vi "test-state-space-util--XXX.vi"() -> (3 "All Tests Passed":bool)   [LabVIEW 2019]
uses:
  <vilib>/Analysis/Matrix/Datatypes/RealMatrix.ctl
  <vilib>/Analysis/baseanly.llb/Real A x B.vi
  <vilib>/Rock Robotics/WPI/ThirdParty/JAS_Junk/TrajLib/MatBuilder_Create.vi
  <vilib>/Analysis/7linalg.llb/Transpose Matrix.vi
  <vilib>/Analysis/7linalg.llb/Real Transpose Matrix.vi
  <vilib>/Rock Robotics/WPI/ThirdParty/JAS_Junk/TrajLib/MatrixHelper_CoerceSize.vi
  <vilib>/Rock Robotics/WPI/ThirdParty/JAS_Junk/TrajLib/Matrix_Ident.vi
  <vilib>/Analysis/Matrix/Numeric/Multiply/Multiply.vi
  <vilib>/Analysis/Matrix/Numeric/Multiply/Multiply - RM,R.vi
  <vilib>/Rock Robotics/WPI/ThirdParty/JAS_Junk/TrajLib/Matrix_Exp.vi
  <vilib>/Rock Robotics/WPI/ThirdParty/JAS_Junk/TrajLib/Matrix_AssignBlock.vi
  <vilib>/Rock Robotics/WPI/ThirdParty/JAS_Junk/TrajLib/Matrix_ExtractFrom.vi
  <vilib>/Analysis/7linalg.llb/Create Special Matrix.vi
  <vilib>/Analysis/7linalg.llb/Create Special Real Matrix.vi
  <vilib>/Analysis/Matrix/Numeric/Add/Add - RM,RM.vi
  <vilib>/Analysis/Matrix/Comparison/Equal/Equal - RM,RM.vi
  <vilib>/Rock Robotics/WPI/ThirdParty/JAS_Junk/TrajLib/Trajectory_Library.lvlib
  <vilib>/Analysis/NI_AALBase.lvlib
  <vilib>/Analysis/Matrix/NI_Matrix.lvlib
panel:
  out "A+B Should be":T1
  out "A + B":T1
  out "Test x passed":bool
  out "Test 3 passed":bool
  out "Test Passed 2":bool
  out "Test Passed 1":bool
  out "Test Passed 0":bool
  out "AQ Passed":bool
  out "AQ - DiscQ":T1
  out "AQ - DiscA":T1
  out "AB-Taylor-Passed":bool
  out "ABTaylor-DiscB":T1
  out "ABTaylor - DiscA":T1
  out "AB-passed":bool
  out "AB-DiscB":T1
  out "AB - DiscA":T1
  out "x1-Disc":T1
  out "DiscA Error":bool
  out "DiscA":T1
  out "Cost Mat":T1
  out "CoVar Mat":T1
  # "1.0,   0.0,    0.0\n\n0.0,     4.0,   0.0, ;\n\n0.0,     0.0,  9.0;"
  # "1.0,      0.0,      0.0, \n\n0.0,   1.0 / 4.0,   0.0, \n\n0.0,       0.0,      1.0 / 9.0,"
  # "VecBuilder.fill(\n          x0.get(0, 0) + 1.0 * x0.get(1, 0), \n          x0.get(1, 0));"
  # "2,\n1"
  # "x0.get(0, 0) + x0.get(1, 0) + 0.5 * u.get(0, 0), \n\nx0.get(0, 0) + u.get(0, 0))"
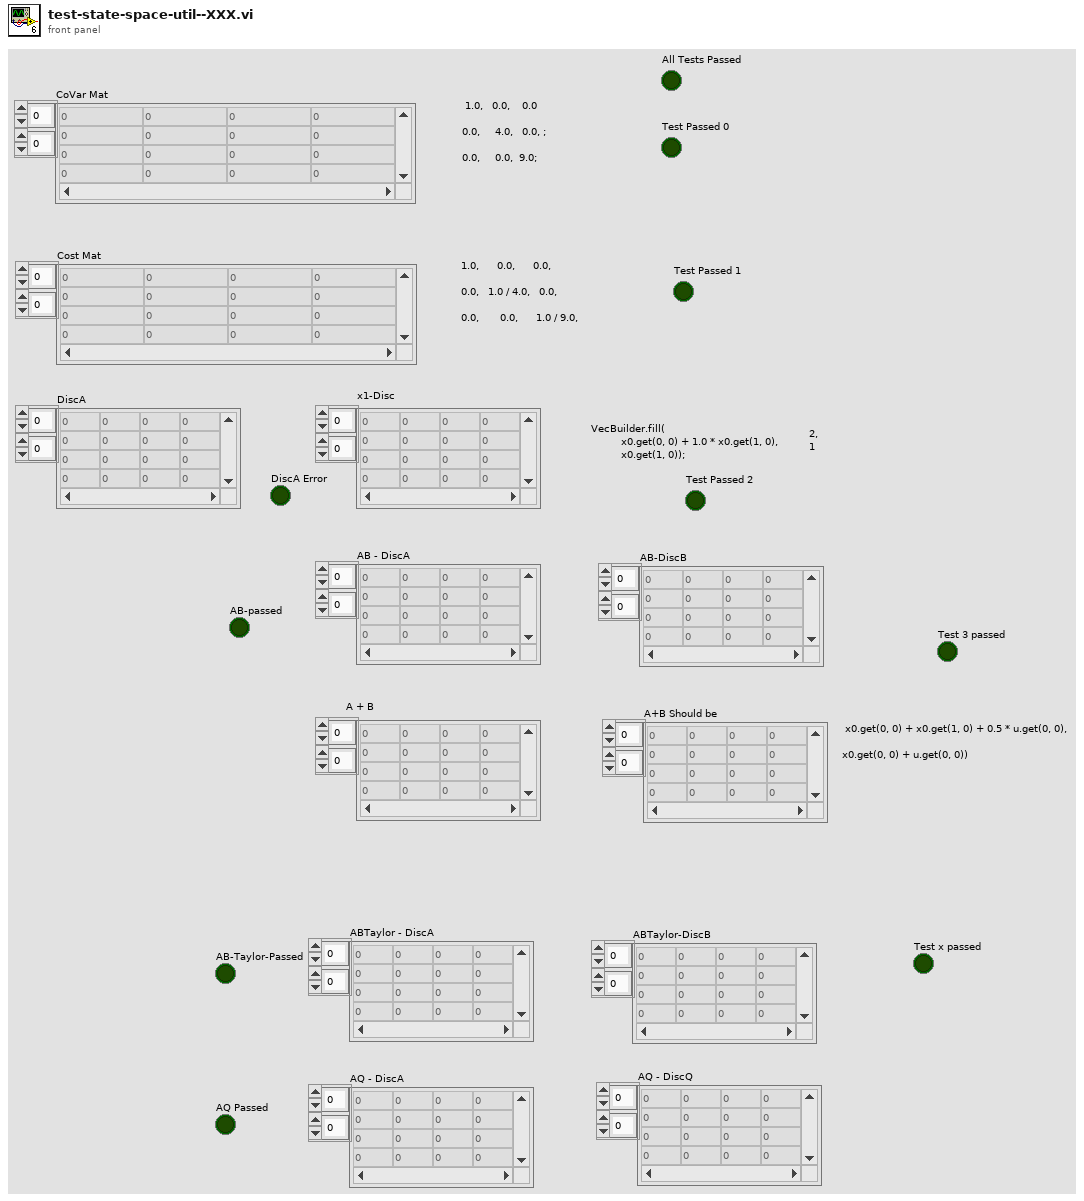
[diagram p1: front panel]
types:
  T1 = typedef "NI_Matrix.lvlib/RealMatrix.ctl" = dbl[][]
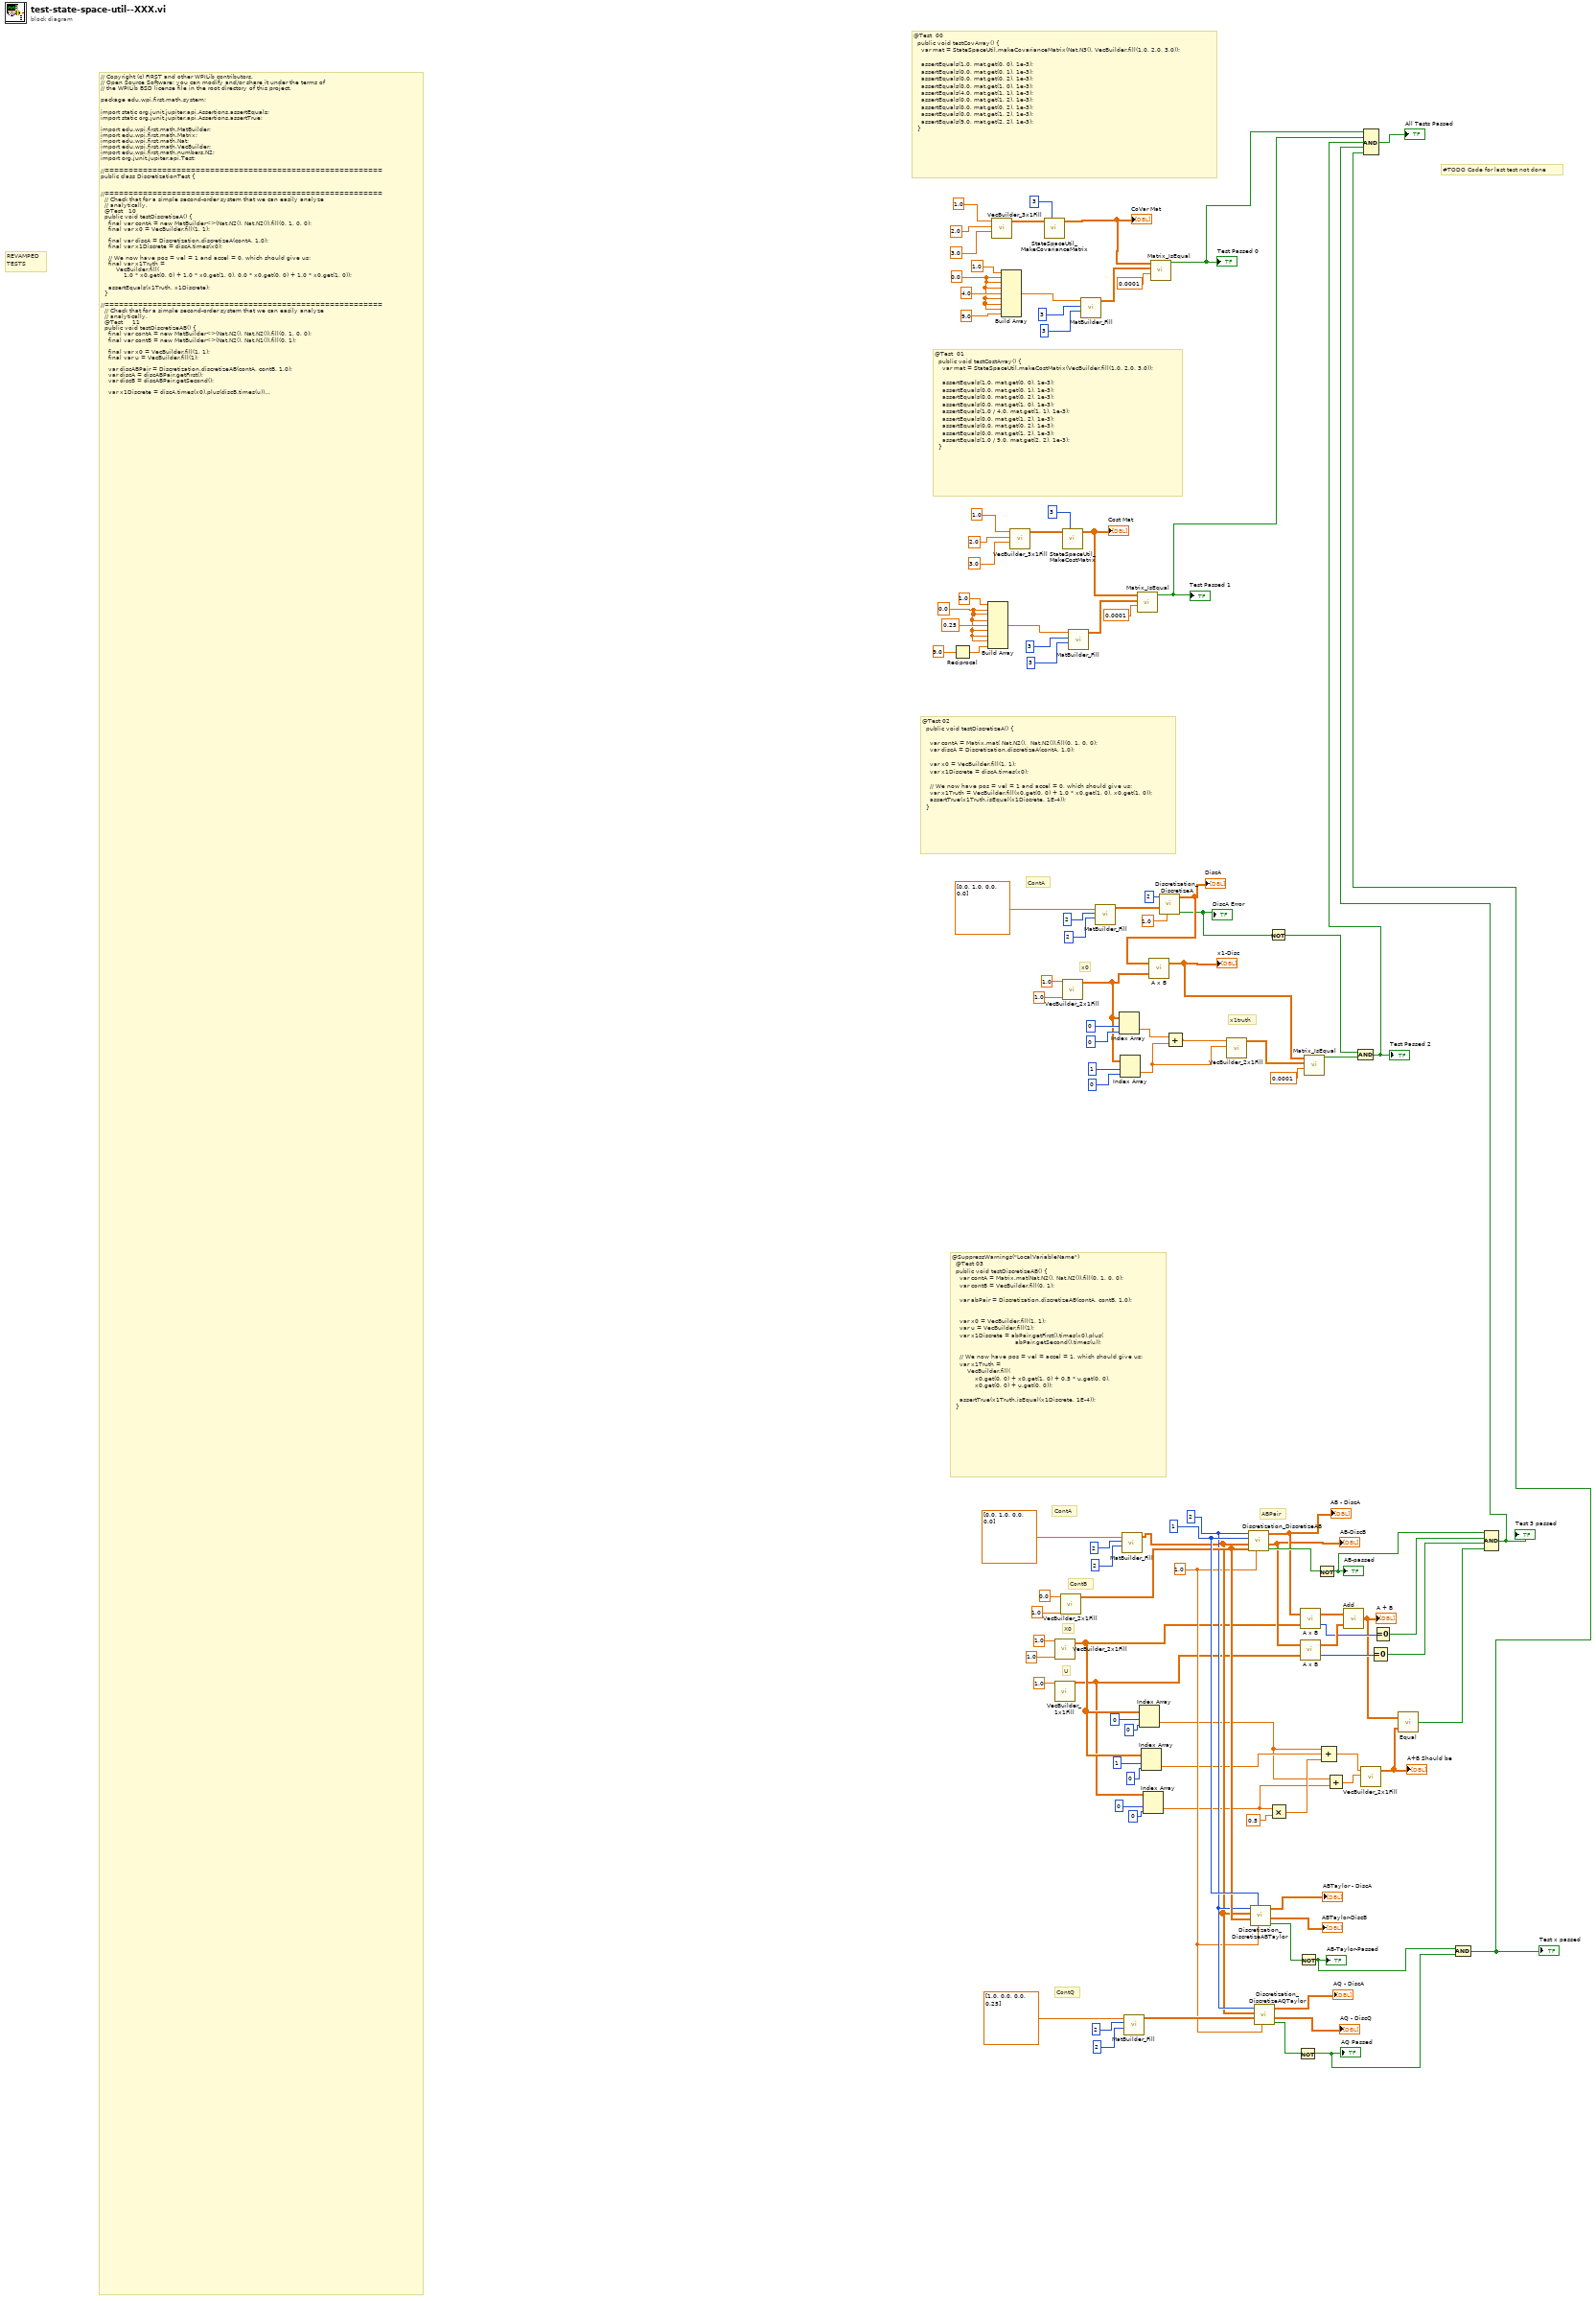
[diagram p0: block diagram]
diagram:
  w61 = 0.0 ("element")
  w71 = 0.0 ("element")
  w79 = 1.0 ("dT_Seconds")
  w89 = 1 ("Inputs")
  w82 = 2 ("States")
  # "REVAMPED\nTESTS"
  # "// Copyright (c) FIRST and other WPILib contributors.\n// Open Source Software; you can modify and/or share it under the terms of\n// the WPILib BSD license file in the root directory of this project.\n\npackage edu.wpi.first.math.system;\n\nimport static org.junit.jupiter.api.Assertions.assertEquals;\nimport static org.junit.jupiter.api.Assertions.assertTrue;\n\nimport edu.wpi.first.math.MatBuilder;\nimport edu.wpi.first.math.Matrix;\nimport edu.wpi.first.math.Nat;\nimport edu.wpi.first.math.VecBuilder;\nimport edu.wpi.first.math.numbers.N2;\nimport org.junit.jupiter.api.Test;\n\n//==========================================================\npublic class DiscretizationTest {\n\n\n//==========================================================\n  // Check that for a simple second-order system that we can easily analyze\n  // analytically,\n  @Test   10\n  public void testDiscretizeA() {\n    final var contA = new MatBuilder<>(Nat.N2(), Nat.N2()).fill(0, 1, 0, 0);\n    final var x0 = VecBuilder.fill(1, 1);\n\n    final var discA = Discretization.discretizeA(contA, 1.0);\n    final var x1Discrete = discA.times(x0);\n\n    // We now have pos = vel = 1 and accel = 0, which should give us:\n    final var x1Truth =\n        VecBuilder.fill(\n            1.0 * x0.get(0, 0) + 1.0 * x0.get(1, 0), 0.0 * x0.get(0, 0) + 1.0 * x0.get(1, 0));\n\n    assertEquals(x1Truth, x1Discrete);\n  }\n\n//==========================================================\n  // Check that for a simple second-order system that we can easily analyze\n  // analytically,\n  @Test     11\n  public void testDiscretizeAB() {\n    final var contA = new MatBuilder<>(Nat.N2(), Nat.N2()).fill(0, 1, 0, 0);\n    final var contB = new MatBuilder<>(Nat.N2(), Nat.N1()).fill(0, 1);\n\n    final var x0 = VecBuilder.fill(1, 1);\n    final var u = VecBuilder.fill(1);\n\n    var discABPair = Discretization.discretizeAB(contA, contB, 1.0);\n    var discA = discABPair.getFirst();\n    var discB = discABPair.getSecond();\n\n    var x1Discrete = discA.times(x0).plus(discB.times(u));\n\n    // We now have pos = vel = accel = 1, which should give us:\n    final var x1Truth =\n        VecBuilder.fill(\n            1.0 * x0.get(0, 0) + 1.0 * x0.get(1, 0) + 0.5 * u.get(0, 0),\n            0.0 * x0.get(0, 0) + 1.0 * x0.get(1, 0) + 1.0 * u.get(0, 0));\n\n    assertEquals(x1Truth, x1Discrete);\n  }\n\n//==========================================================\n  //                                             dt\n  // Test that the discrete approximation of Q ˜ ? e^(At) Q e^(A?t) dt\n  //                                             0\n  @Test    12\n  public void testDiscretizeSlowModelAQ() {\n    final var contA = new MatBuilder<>(Nat.N2(), Nat.N2()).fill(0, 1, 0, 0);\n    final var contQ = new MatBuilder<>(Nat.N2(), Nat.N2()).fill(1, 0, 0, 1);\n\n    final double dt = 1.0;\n\n    final var discQIntegrated =\n        RungeKuttaTimeVarying.rungeKuttaTimeVarying(\n            (Double t, Matrix<N2, N2> x) ->\n                contA.times(t).exp().times(contQ).times(contA.transpose().times(t).exp()),\n            0.0,\n            new Matrix<>(Nat.N2(), Nat.N2()),\n            dt);\n\n    var discAQPair = Discretization.discretizeAQ(contA, contQ, dt);\n    var discQ = discAQPair.getSecond();\n\n    assertTrue(\n        discQIntegrated.minus(discQ).normF() < 1e-10,\n        \"Expected these to be nearly equal:\\ndiscQ:\\n\"\n            + discQ\n            + \"\\ndiscQIntegrated:\\n\"\n            + discQIntegrated);\n  }\n\n//==========================================================\n  //                                             dt\n  // Test that the discrete approximation of Q ˜ ? e^(At) Q e^(A?t) dt\n  //                                             0\n  @Test\n  public void testDiscretizeFastModelAQ() {\n    final var contA = new MatBuilder<>(Nat.N2(), Nat.N2()).fill(0, 1, 0, -1406.29);\n    final var contQ = new MatBuilder<>(Nat.N2(), Nat.N2()).fill(0.0025, 0, 0, 1);\n\n    final var dt = 0.005;\n\n    final var discQIntegrated =\n        RungeKuttaTimeVarying.rungeKuttaTimeVarying(\n            (Double t, Matrix<N2, N2> x) ->\n                contA.times(t).exp().times(contQ).times(contA.transpose().times(t).exp()),\n            0.0,\n            new Matrix<>(Nat.N2(), Nat.N2()),\n            dt);\n\n    var discAQPair = Discretization.discretizeAQ(contA, contQ, dt);\n    var discQ = discAQPair.getSecond();\n\n    assertTrue(\n        discQIntegrated.minus(discQ).normF() < 1e-3,\n        \"Expected these to be nearly equal:\\ndiscQ:\\n\"\n            + discQ\n            + \"\\ndiscQIntegrated:\\n\"\n            + discQIntegrated);\n  }\n\n//==========================================================\n  // Test that the Taylor series discretization produces nearly identical results.\n  @Test\n  public void testDiscretizeSlowModelAQTaylor() {\n    final var contA = new MatBuilder<>(Nat.N2(), Nat.N2()).fill(0, 1, 0, 0);\n    final var contQ = new MatBuilder<>(Nat.N2(), Nat.N2()).fill(1, 0, 0, 1);\n\n    final var dt = 1.0;\n\n    // Continuous Q should be positive semidefinite\n    final var esCont = contQ.getStorage().eig();\n    for (int i = 0; i < contQ.getNumRows(); ++i) {\n      assertTrue(esCont.getEigenvalue(i).real >= 0);\n    }\n\n    final var discQIntegrated =\n        RungeKuttaTimeVarying.rungeKuttaTimeVarying(\n            (Double t, Matrix<N2, N2> x) ->\n                contA.times(t).exp().times(contQ).times(contA.transpose().times(t).exp()),\n            0.0,\n            new Matrix<>(Nat.N2(), Nat.N2()),\n            dt);\n\n    var discA = Discretization.discretizeA(contA, dt);\n\n    var discAQPair = Discretization.discretizeAQ(contA, contQ, dt);\n    var discATaylor = discAQPair.getFirst();\n    var discQTaylor = discAQPair.getSecond();\n\n    assertTrue(\n        discQIntegrated.minus(discQTaylor).normF() < 1e-10,\n        \"Expected these to be nearly equal:\\ndiscQTaylor:\\n\"\n            + discQTaylor\n            + \"\\ndiscQIntegrated:\\n\"\n            + discQIntegrated);\n    assertTrue(discA.minus(discATaylor).normF() < 1e-10);\n\n    // Discrete Q should be positive semidefinite\n    final var esDisc = discQTaylor.getStorage().eig();\n    for (int i = 0; i < discQTaylor.getNumRows(); ++i) {\n      assertTrue(esDisc.getEigenvalue(i).real >= 0);\n    }\n  }\n\n//==========================================================\n  // Test that the Taylor series discretization produces nearly identical results.\n  @Test\n  public void testDiscretizeFastModelAQTaylor() {\n    final var contA = new MatBuilder<>(Nat.N2(), Nat.N2()).fill(0, 1, 0, -1500);\n    final var contQ = new MatBuilder<>(Nat.N2(), Nat.N2()).fill(0.0025, 0, 0, 1);\n\n    final var dt = 0.005;\n\n    // Continuous Q should be positive semidefinite\n    final var esCont = contQ.getStorage().eig();\n    for (int i = 0; i < contQ.getNumRows(); ++i) {\n      assertTrue(esCont.getEigenvalue(i).real >= 0);\n    }\n\n    final var discQIntegrated =\n        RungeKuttaTimeVarying.rungeKuttaTimeVarying(\n            (Double t, Matrix<N2, N2> x) ->\n                contA.times(t).exp().times(contQ).times(contA.transpose().times(t).exp()),\n            0.0,\n            new Matrix<>(Nat.N2(), Nat.N2()),\n            dt);\n\n    var discA = Discretization.discretizeA(contA, dt);\n\n    var discAQPair = Discretization.discretizeAQ(contA, contQ, dt);\n    var discATaylor = discAQPair.getFirst();\n    var discQTaylor = discAQPair.getSecond();\n\n    assertTrue(\n        discQIntegrated.minus(discQTaylor).normF() < 1e-3,\n        \"Expected these to be nearly equal:\\ndiscQTaylor:\\n\"\n            + discQTaylor\n            + \"\\ndiscQIntegrated:\\n\"\n            + discQIntegrated);\n    assertTrue(discA.minus(discATaylor).normF() < 1e-10);\n\n    // Discrete Q should be positive semidefinite\n    final var esDisc = discQTaylor.getStorage().eig();\n    for (int i = 0; i < discQTaylor.getNumRows(); ++i) {\n      assertTrue(esDisc.getEigenvalue(i).real >= 0);\n    }\n  }\n\n//==========================================================\n  // Test that DiscretizeR() works\n  @Test\n  public void testDiscretizeR() {\n    var contR = Matrix.mat(Nat.N2(), Nat.N2()).fill(2.0, 0.0, 0.0, 1.0);\n    var discRTruth = Matrix.mat(Nat.N2(), Nat.N2()).fill(4.0, 0.0, 0.0, 2.0);\n\n    var discR = Discretization.discretizeR(contR, 0.5);\n\n    assertTrue(\n        discRTruth.minus(discR).normF() < 1e-10,\n        \"Expected these to be nearly equal:\\ndiscR:\\n\" + discR + \"\\ndiscRTruth:\\n\" + discRTruth);\n  }\n}"
  # "U"
  # "X0"
  # "ContB"
  # "ABPair"
  # "#TODO Code for last test not done"
  # "x1truth"
  # "x0"
  # "ContQ"
  # "ContA"
  # "@SuppressWarnings(\"LocalVariableName\")\n  @Test 03\n  public void testDiscretizeAB() {\n    var contA = Matrix.mat(Nat.N2(), Nat.N2()).fill(0, 1, 0, 0);\n    var contB = VecBuilder.fill(0, 1);\n\n    var abPair = Discretization.discretizeAB(contA, contB, 1.0);\n\n\n    var x0 = VecBuilder.fill(1, 1);\n    var u = VecBuilder.fill(1);\n    var x1Discrete = abPair.getFirst().times(x0).plus(\n                                 abPair.getSecond().times(u));\n\n    // We now have pos = vel = accel = 1, which should give us:\n    var x1Truth =\n        VecBuilder.fill(\n            x0.get(0, 0) + x0.get(1, 0) + 0.5 * u.get(0, 0), \n            x0.get(0, 0) + u.get(0, 0));\n\n    assertTrue(x1Truth.isEqual(x1Discrete, 1E-4));\n  }"
  # "ContA"
  # "@Test 02\n  public void testDiscretizeA() {\n\n    var contA = Matrix.mat( Nat.N2(),  Nat.N2()).fill(0, 1, 0, 0);\n    var discA = Discretization.discretizeA(contA, 1.0);\n\n    var x0 = VecBuilder.fill(1, 1);\n    var x1Discrete = discA.times(x0);\n\n    // We now have pos = vel = 1 and accel = 0, which should give us:\n    var x1Truth = VecBuilder.fill(x0.get(0, 0) + 1.0 * x0.get(1, 0), x0.get(1, 0));\n    assertTrue(x1Truth.isEqual(x1Discrete, 1E-4));\n  }"
  # "@Test  01\n  public void testCostArray() {\n    var mat = StateSpaceUtil.makeCostMatrix(VecBuilder.fill(1.0, 2.0, 3.0));\n\n    assertEquals(1.0, mat.get(0, 0), 1e-3);\n    assertEquals(0.0, mat.get(0, 1), 1e-3);\n    assertEquals(0.0, mat.get(0, 2), 1e-3);\n    assertEquals(0.0, mat.get(1, 0), 1e-3);\n    assertEquals(1.0 / 4.0, mat.get(1, 1), 1e-3);\n    assertEquals(0.0, mat.get(1, 2), 1e-3);\n    assertEquals(0.0, mat.get(0, 2), 1e-3);\n    assertEquals(0.0, mat.get(1, 2), 1e-3);\n    assertEquals(1.0 / 9.0, mat.get(2, 2), 1e-3);\n  }"
  # "@Test  00\n  public void testCovArray() {\n    var mat = StateSpaceUtil.makeCovarianceMatrix(Nat.N3(), VecBuilder.fill(1.0, 2.0, 3.0));\n\n    assertEquals(1.0, mat.get(0, 0), 1e-3);\n    assertEquals(0.0, mat.get(0, 1), 1e-3);\n    assertEquals(0.0, mat.get(0, 2), 1e-3);\n    assertEquals(0.0, mat.get(1, 0), 1e-3);\n    assertEquals(4.0, mat.get(1, 1), 1e-3);\n    assertEquals(0.0, mat.get(1, 2), 1e-3);\n    assertEquals(0.0, mat.get(0, 2), 1e-3);\n    assertEquals(0.0, mat.get(1, 2), 1e-3);\n    assertEquals(9.0, mat.get(2, 2), 1e-3);\n  }"
  n1 = Reciprocal(x=9.0 ("element")) -> (1/x=w57:dbl)
  n2 = Build Array(1.0 ("element"), w61, w61, w61, 0.25 ("element"), w61, w61, w61, w57) -> (w64:dbl[])
  n3 = call <vilib>:"VecBuilder_3x1Fill.vi"("R2"=3.0, "R1"=2.0, "R0"=1.0) -> ("output matrix"=w110:T1)  [unwired: 8 in]
  n4 = Build Array(1.0 ("element"), w71, w71, w71, 4.0 ("element"), w71, w71, w71, 9.0 ("element")) -> (w74:dbl[])
  n5 = call <vilib>:"VecBuilder_3x1Fill.vi"("R2"=3.0, "R1"=2.0, "R0"=1.0) -> ("output matrix"=w105:T1)  [unwired: 8 in]
  n6 = call <vilib>:"StateSpaceUtil_MakeCovarianceMatrix.vi"("States"=3, "StdDevs"=w110) -> ("Covariance Matrix"=w69:T1)  [unwired: 8 in, 1 out]
  "CoVar Mat" <- w69
  n7 = call <vilib>:"VecBuilder_2x1Fill.vi"("R1"=1.0, "R0"=1.0 ("R0_C0")) -> ("output matrix"=w12:T1)  [unwired: 9 in]
  n8 = call <vilib>:"VecBuilder_1x1Fill.vi"("R0_C0"=1.0) -> ("output matrix"=w11:T1)  [unwired: 10 in]
  n9 = call <vilib>:"VecBuilder_2x1Fill.vi"("R1"=1.0, "R0"=0.0 ("R0_C0")) -> ("output matrix"=w88:T1)  [unwired: 9 in]
  n10 = call <vilib>:"StateSpaceUtil_MakeCostMatrix.vi"("States"=3, "Costs"=w105) -> ("Costs Matrix"=w56:T1)  [unwired: 8 in, 1 out]
  "Cost Mat" <- w56
  n11 = call <vilib>:"VecBuilder_2x1Fill.vi"("R1"=1.0, "R0"=1.0 ("R0_C0")) -> ("output matrix"=w50:T1)  [unwired: 9 in]
  n12 = call <vilib>:"MatBuilder_Fill.vi"("Columns"=3, "Rows"=3, "Value List"=w64) -> ("output matrix"=w60:T1)  [unwired: 8 in]
  n13 = call <vilib>:"MatBuilder_Fill.vi"("Columns"=3, "Rows"=3, "Value List"=w74) -> ("output matrix"=w68:T1)  [unwired: 8 in]
  n14 = call <vilib>:"MatBuilder_Fill.vi"("Columns"=2, "Rows"=2, "Value List"=dbl[] [0.0, 1.0, 0.0, 0.0]) -> ("output matrix"=w98:T1)  [unwired: 8 in]
  n15 = Index Array(array=w50, index (row)=0, index (col)=0) -> (element=w49:dbl)
  n16 = Index Array(array=w50, index (row)=1, index (col)=0) -> (element=w47:dbl)
  n17 = call <vilib>:"MatBuilder_Fill.vi"("Columns"=2, "Rows"=2, "Value List"=dbl[] [0.0, 1.0, 0.0, 0.0]) -> ("output matrix"=w81:T1)  [unwired: 8 in]
  n18 = call <vilib>:"MatBuilder_Fill.vi"("Columns"=2, "Rows"=2, "Value List"=dbl[] [1.0, 0.0, 0.0, 0.25]) -> ("output matrix"=w80:T1)  [unwired: 8 in]
  n19 = call <vilib>:"Matrix_IsEqual.vi"("Tolerance"=0.0001, "other"=w60, "input matrix"=w56) -> ("Equal"=w40:bool)  [unwired: 8 in]
  "Test Passed 1" <- w40
  n20 = Index Array(array=w12, index (row)=0, index (col)=0) -> (element=w5:dbl)
  n21 = Index Array(array=w12, index (row)=1, index (col)=0) -> (element=w9:dbl)
  n22 = Index Array(array=w11, index (row)=0, index (col)=0) -> (element=w4:dbl)
  n23 = call <vilib>:"Matrix_IsEqual.vi"("Tolerance"=0.0001, "other"=w68, "input matrix"=w69) -> ("Equal"=w41:bool)  [unwired: 8 in]
  "Test Passed 0" <- w41
  n24 = call <vilib>:"Discretization_DiscretizeA.vi"("dT_Seconds"=1.0, "ContA"=w98, "States"=2) -> ("Error"=w43:bool, "DiscA"=w95:T1)  [unwired: 7 in]
  "DiscA" <- w95
  "DiscA Error" <- w43
  n25 = call-poly <vilib>:"A x B.vi"("B"=w50, "A"=w95) -> ("A x B"=w46:T1)  [unwired: 1 out]
  "x1-Disc" <- w46
  n26 = Add(x=w49, y=w47) -> (x+y=w48:dbl)
  n27 = call <vilib>:"VecBuilder_2x1Fill.vi"("R1"=w47, "R0"=w48) -> ("output matrix"=w45:T1)  [unwired: 9 in]
  n28 = call <vilib>:"Discretization_DiscretizeAB.vi"("dT_Seconds"=w79, "ContB"=w88, "ContA"=w81, "Inputs"=w89, "States"=w82) -> ("Error"=w37:bool, "DiscB"=w27:T1, "DiscA"=w31:T1)  [unwired: 4 in]
  "AB - DiscA" <- w31
  "AB-DiscB" <- w27
  n29 = call <vilib>:"Discretization_DiscretizeABTaylor.vi"("dT_Seconds"=w79, "Inputs"=w89, "ContB"=w88, "ContA"=w81, "States"=w82) -> ("Error"=w36:bool, "DiscB"=→"ABTaylor-DiscB":T1, "DiscA"=→"ABTaylor - DiscA":T1)  [unwired: 4 in]
  n30 = call <vilib>:"Discretization_DiscretizeAQTaylor.vi"("dT_Seconds"=w79, "ContQ"=w80, "ContA"=w81, "States"=w82) -> ("Error"=w34:bool, "DiscQ"=→"AQ - DiscQ":T1, "DiscA"=→"AQ - DiscA":T1)  [unwired: 5 in]
  n31 = Not(x=w43) -> (.not. x?=w42:bool)
  n32 = Multiply(x=w4, y=0.5) -> (x*y=w8:dbl)
  n33 = Not(x=w34) -> (.not. x?=w32:bool)
  "AQ Passed" <- w32
  n34 = Not(x=w36) -> (.not. x?=w33:bool)
  "AB-Taylor-Passed" <- w33
  n35 = call-poly <vilib>:"A x B.vi"("B"=w11, "A"=w27) -> ("error"=w23:i32, "A x B"=w25:T1)
  n36 = call-poly <vilib>:"A x B.vi"("B"=w12, "A"=w31) -> ("error"=w24:i32, "A x B"=w26:T1)
  n37 = call <vilib>:"Matrix_IsEqual.vi"("Tolerance"=0.0001, "other"=w45, "input matrix"=w46) -> ("Equal"=w44:bool)  [unwired: 8 in]
  n38 = Not(x=w37) -> (.not. x?=w35:bool)
  "AB-passed" <- w35
  n39 = Compound Arithmetic op=ADD(w5, w9, w8) -> (w7:dbl)
  n40 = Add(x=w5, y=w4) -> (x+y=w6:dbl)
  n41 = call-poly <vilib>:"Add.vi"("Real Matrix B"=w25, "Real Matrix A"=w26) -> ("A + B"=w2:T1)
  "A + B" <- w2
  n42 = Compound Arithmetic op=AND(w42, w44) -> (w39:bool)
  "Test Passed 2" <- w39
  n43 = call <vilib>:"VecBuilder_2x1Fill.vi"("R1"=w6, "R0"=w7) -> ("output matrix"=w3:T1)  [unwired: 9 in]
  "A+B Should be" <- w3
  n44 = Equal To 0?(x=w23) -> (x = 0?=w21:bool)
  n45 = Equal To 0?(x=w24) -> (x = 0?=w22:bool)
  n46 = call-poly <vilib>:"Equal.vi"("Real Matrix B"=w3, "Real Matrix A"=w2) -> ("A = B?"=w1:bool)
  n47 = Compound Arithmetic op=AND(w33, w32) -> (w19:bool)
  "Test x passed" <- w19
  n48 = Compound Arithmetic op=AND(w35, w22, w21, w1) -> (w20:bool)
  "Test 3 passed" <- w20
  n49 = Compound Arithmetic op=AND(w41, w40, w39, w20, w19) -> (→"All Tests Passed":bool)
